vi "example_2.vi"(8 "Error In":errorcluster) -> (0 "Error Out":errorcluster)   [LabVIEW 2014]
panel:
  in  "cyclesCnt":i32=42
  out "number out":i32
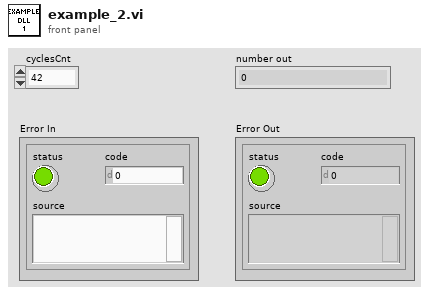
[diagram p1: front panel]
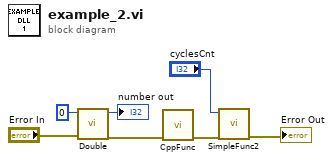
[diagram p0: block diagram]
diagram:
  n1 = call "Double.vi"("Error In"="Error In", "number in"=0) -> ("Error Out"=w4:errorcluster, "number out"=→"number out":i32)  [unwired: 8 in]
  n2 = call "CppFunc.vi"("Error In"=w4) -> ("Error Out"=w3:errorcluster)  [unwired: 10 in]
  n3 = call "SimpleFunc2.vi"("Error In"=w3, "cyclesCnt"="cyclesCnt") -> ("Error Out"=→"Error Out":errorcluster)  [unwired: 9 in]
